vi "FGGA_Scroll_Pump_interface_server.vi"() -> ()   [LabVIEW 2014]
uses:
  <vilib>/NI/STM/TCP/TCP Write Options.ctl
  C:/Program Files (x86)/National Instruments/LabVIEW 2014/examples/Data Communication/Network Streams/Simple Network Streams/support/Network Stream Command.ctl
  <vilib>/Instr/_visa.llb/VISA Set IO Buffer Mask.ctl
  <vilib>/Platform/TimedLoop/XDataNode/timing_clust.ctl
  <vilib>/Platform/TimedLoop/XDataNode/nitl_modes.ctl
  <vilib>/Platform/TimedLoop/XDataNode/wakeup.ctl
  <vilib>/NI/STM/SubVIs/MetaDataElement.ctl
  <vilib>/NI/STM/TCP/Write Meta Data (TCP Ref).vi
  <vilib>/NI/STM/TCP/Get Connection Reference (TCP).vi
  <vilib>/Instr/_visa.llb/VISA Configure Serial Port (Instr).vi
  <vilib>/NI/STM/TCP/Write Meta Data (TCP Clst).vi
  <vilib>/NI/STM/TCP/Write Message (TCP).vi
  <vilib>/platform/TimedLoop/XDataNode/XDataNode.xnode
  <vilib>/Platform/TimedLoop/XDataNode/XDNodeRunTimeDep.lvlib
  <vilib>/NI/STM/NI STM.lvlib
panel:
  in  "options":T1={"ignore timeout error"=FALSE, "timeout ms (1000)"=1000}
  out "Standby Speed %\nDefault Set Value":u32=66 min=66 max=100
  out "error out 3":errorcluster
  out "Message Receive Array":string[](array[string])
  out "Scroll pump\nCommand":string[](array[string])
  out "Network Stream Error":errorcluster
  out "Standby Speed threshold":u32(slide) scale=66.0..100.0
  out "Normal Speed threshold":u32(slide) scale=50.0..100.0
  out "running?":bool
  out "Loop Count":i32
  in  "stop":bool
  out "Use Standby Speed":bool
  out "Serial / Pump Power cut error out":errorcluster
  in  "VISA resource name":refnum<visa-resource-name>="ASRL10::INSTR"
  out "Pump On/Off":bool
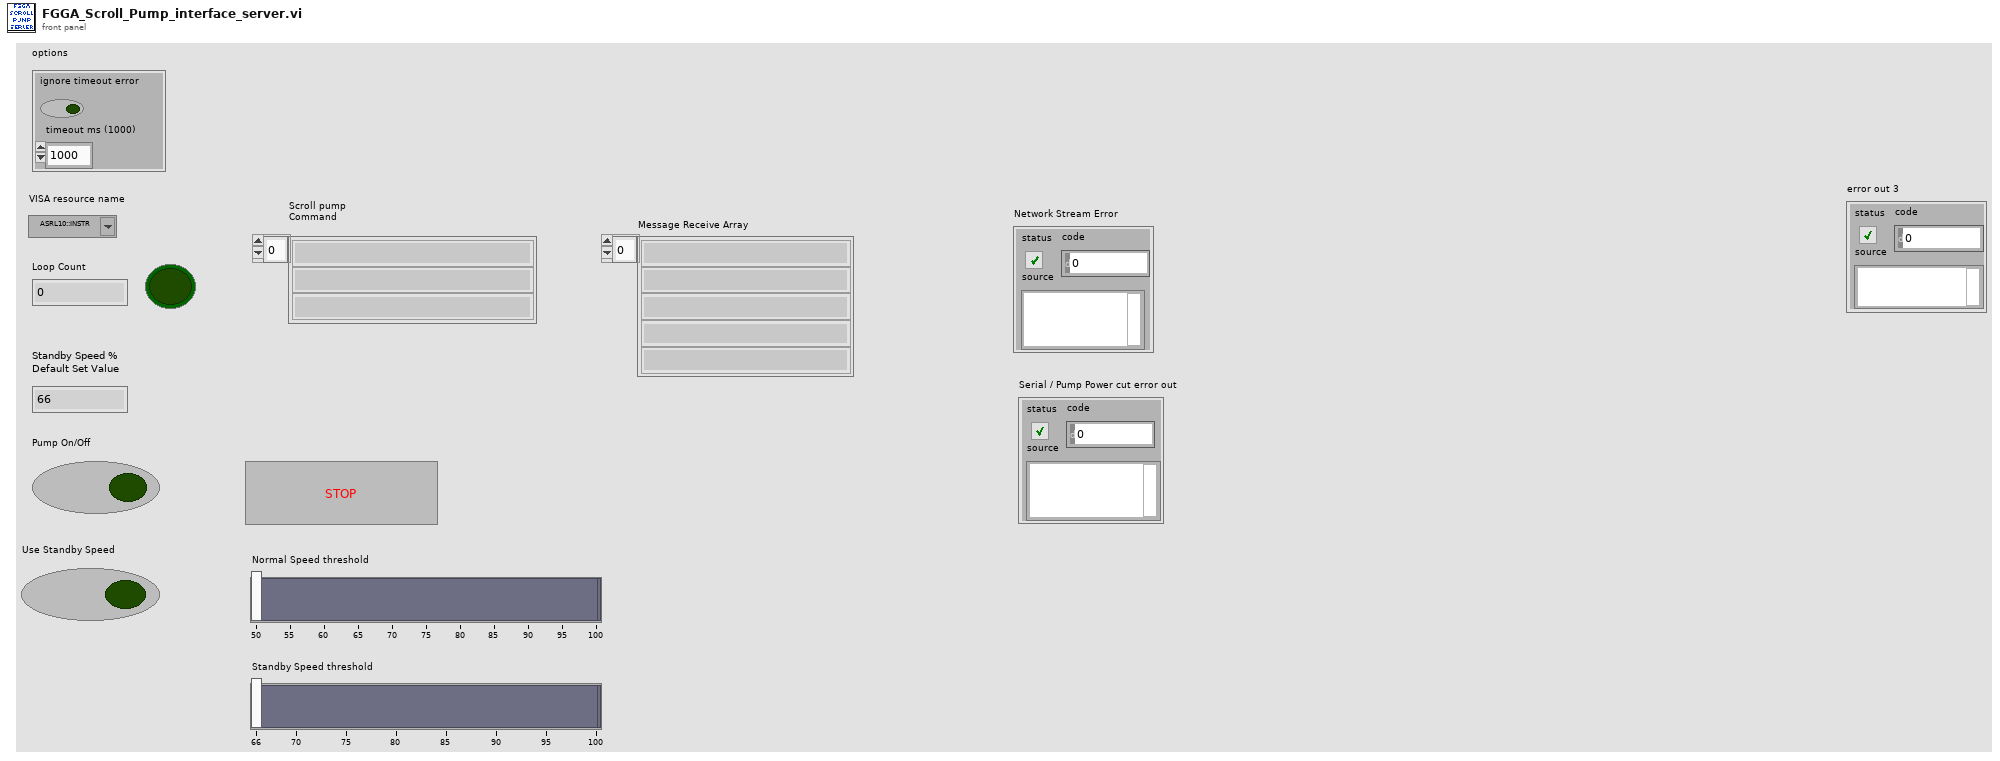
[diagram p1: front panel]
types:
  T1 = typedef "NI STM.lvlib/TCP Write Options.ctl" = cluster{"ignore timeout error":bool, "timeout ms (1000)":i32}
  T2 = typedef "XDNodeRunTimeDep.lvlib/timing_clust.ctl" = cluster{"Expected End [f-1]":u64, "Actual End [f-1]":u64, "Finished Late? [f-1]":bool, "Expected End [i-1]":u64, "Actual End [i-1]":u64, "Finished Late? [i-1]":bool, "Expected Start [i]":u64, "Actual Start [i]":u64, "Expected Start [f]":u64, "Actual Start [f]":u64, "Source Name":string, "Structure Name":string, "Period":i64, "Deadline":i64, "Offset":i64, "Start":i64, "Priority":i32, "Timeout":i32, "Mode":T3, "Wakeup Reason":T4, "Error":errorcluster, "Source Type":string, "Secondary Source Type":string, "Global End Time":u64, "Global Start Time":u64, "Frame Duration":u64, "Iteration Duration":u64, "Assigned CPU":i32, "I/O Scan Engine Mode":u32}
  T3 = typedef "XDNodeRunTimeDep.lvlib/nitl_modes.ctl" = enum32{"No Change", "Process missed periods, maintain original phase", "Discard missed periods, maintain original phase", "Process missed periods, ignore original phase", "Discard missed periods, ignore original phase"}
  T4 = typedef "XDNodeRunTimeDep.lvlib/wakeup.ctl" = enum32{"Normal", "Aborted", "Asynchronous wakeup", "Timing source error", "Timed loop error", "Timeout"}
  T5 = typedef "VISA Set IO Buffer Mask.ctl" = u16
  T6 = typedef "NI STM.lvlib/MetaDataElement.ctl" = string
  T7 = typedef "NI STM.lvlib/TCP Connection Info.ctl" = cluster{"connection ID":refnum<k5>, "meta data":T6[]}
  T8 = typedef "Network Stream Command.ctl" = cluster{"Message":string, "Message Data":variant}
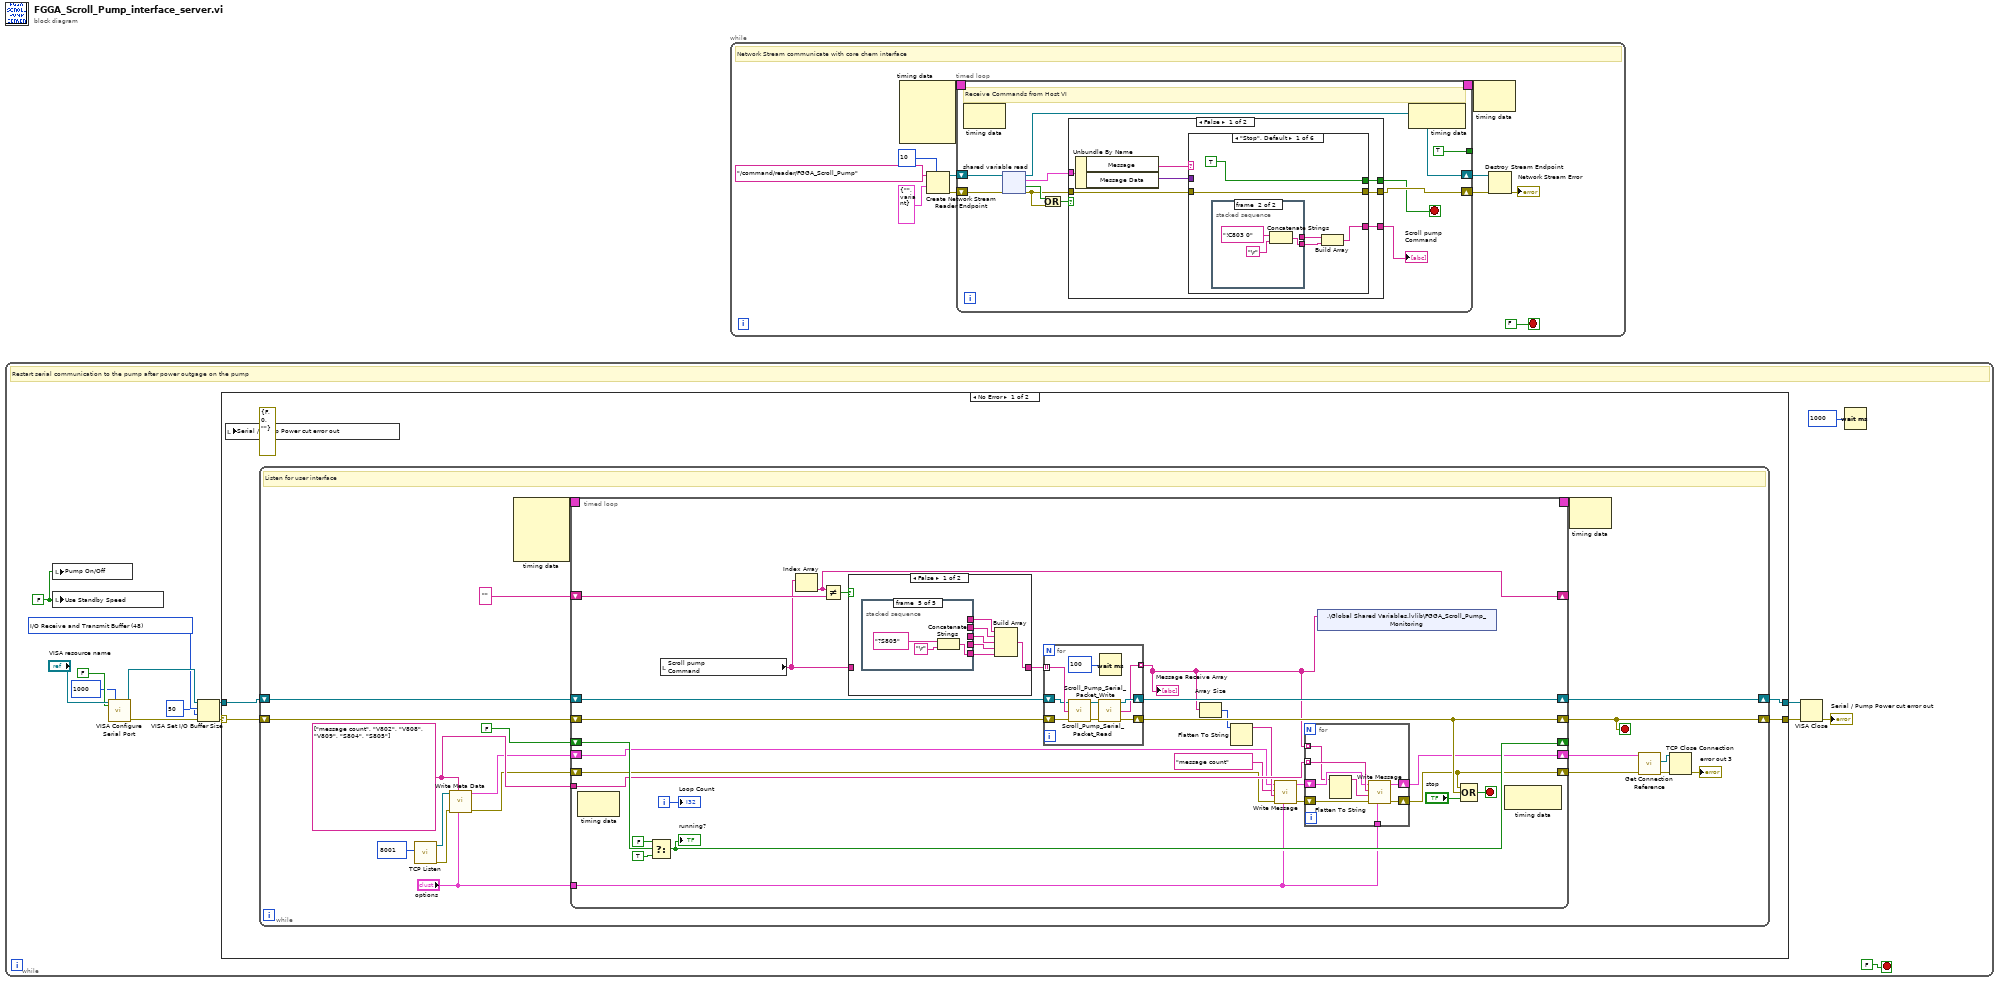
[diagram p0: block diagram]
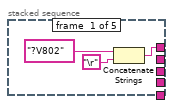
[diagram p2: hidden frame]
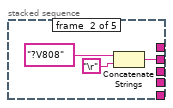
[diagram p3: hidden frame]
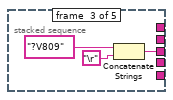
[diagram p4: hidden frame]
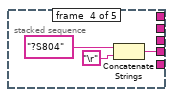
[diagram p5: hidden frame]
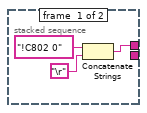
[diagram p8: hidden frame]
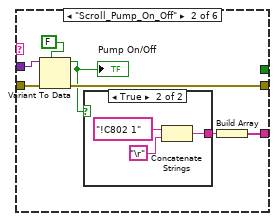
[diagram p9: hidden frame]
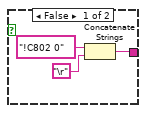
[diagram p10: hidden frame]
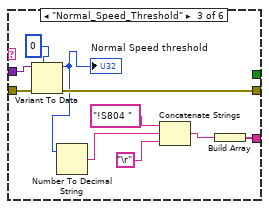
[diagram p11: hidden frame]
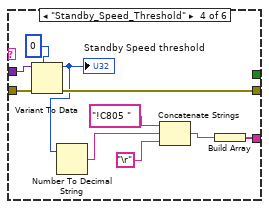
[diagram p12: hidden frame]
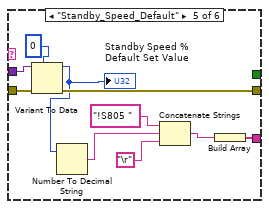
[diagram p13: hidden frame]
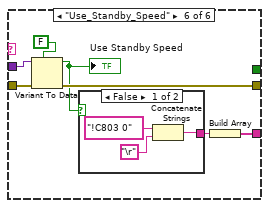
[diagram p14: hidden frame]
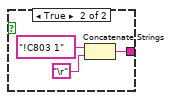
[diagram p15: hidden frame]
diagram:
  n1 = while {
    stop <- FALSE stop-if-true
    w2 = FALSE
    w11 = T5 48 items=["I/O Receive Buffer"=16, "I/O Transmit Buffer"=32, "I/O Receive and Transmit Buffer"=48] ("Mask")
    # "Restart serial communication to the pump after power outgage on the pump"
    n2 = local write "Pump On/Off"(w2) -> ()
    n3 = local write "Use Standby Speed"(w2) -> ()
    n4 = call-poly "VISA Configure Serial Port"("VISA resource name"="VISA resource name", "timeout (10sec)"=u32 1000, "Enable Termination\nChar (T)"=FALSE ("Enable Termination\nChar (T)")) -> ("VISA resource name out"=w12:refnum<visa-resource-name>, "error out"=w13:errorcluster)  [unwired: 11 in]
    n5 = VISA Set I/O Buffer Size(VISA resource name=w12, mask (16)=w11, size (4096)=u32 50, error in (no error)=w13) -> (VISA resource name out=w5:refnum<visa-resource-name>, error out=w4:errorcluster)
    n6 = case shown="No Error" w4 {
      selector: w4 -> [w20 w112]
      tunnel: w5 -> [w19 w113]
      tunnel: [w16 w113] -> w8
      tunnel: [w18 w112] -> w7
      frame No Error {
        n7 = local write "Serial / Pump Power cut error out"(errorcluster {"status"=FALSE, "code"=0, "source"=""} ("error out 2")) -> ()
        n8 = while {
          shift-right: [w22] -> w18
          shift-left: w20 -> [w37]
          shift-right: [w23] -> w16
          shift-left: w19 -> [w36]
          stop <- w22 stop-if-true
          w31 = T6[] ["message count", "V802", "V808", "V809", "S804", "S805"] ("meta data")
          # "Listen for user interface"
          n9 = call <vilib>:"TCP Listen.vi"("port"=u16 8001) -> ("error out"=w32:errorcluster, "connection ID"=w33:refnum<k5>)  [unwired: 6 in, 3 out]
          n10 = call-poly <vilib>:"Write Meta Data.vi"("options"="options", "meta data"=w31, "error in"=w32, "connection ID"=w33) -> ("error out"=w29:errorcluster, "connection info out"=w30:T7)  [unwired: 1 in, 5 out]
          n11 = node-c288() -> (w40:T2)  [unwired: 4 in]
          n12 = timed-loop {
            shift-right: [w64] -> _
            shift-left: FALSE -> [w67]
            shift-right: [w54] -> _
            shift-left: "" -> [w60]
            timing: w40 -> [_]
            timing-out: [_] -> w39
            tunnel: w31 -> [w53]
            shift-right: [w51] -> w23
            shift-left: w36 -> [w56]
            shift-right: [w62] -> w22
            shift-left: w37 -> [w55]
            shift-right: [w52] -> w25
            shift-left: w30 -> [w47]
            shift-right: [w50] -> w24
            shift-left: w29 -> [w48]
            tunnel: "options" -> [w41]
            i -> [w68]
            stop <- w61 stop-if-true
            n13 = node-c288() -> ()  [unwired: 1 in, 1 out]
            n14 = Select(t=FALSE, s=w67, f=TRUE) -> (s? t:f=w64:bool)
            "running?" <- w64
            n15 = local read "Scroll pump\nCommand"() -> (w58:string[])
            n16 = Index Array(array=w58) -> (element=w54:string)  [unwired: 1 in]
            n17 = Not Equal?(x=w54, y=w60) -> (x != y?=w59:bool)
            n18 = case shown="False" w59 {
              tunnel: [w81 w100] -> w57
              tunnel: w58 -> [_ w100]
              frame False {
                n19 = stacked-sequence {
                  tunnel: [w85 _ _ _ _] -> w82
                  tunnel: [_ w88 _ _ _] -> w83
                  tunnel: [_ _ w91 _ _] -> w84
                  tunnel: [_ _ _ w94 _] -> w80
                  tunnel: [_ _ _ _ w97] -> w79
                  frame #0 {
                    n20 = Concatenate Strings("?V802" ("string"), "\r") -> (w85:string)
                  }
                  frame #1 {
                    n21 = Concatenate Strings("?V808" ("string"), "\r") -> (w88:string)
                  }
                  frame #2 {
                    n22 = Concatenate Strings("?V809" ("string"), "\r") -> (w91:string)
                  }
                  frame #3 {
                    n23 = Concatenate Strings("?S804" ("string"), "\r") -> (w94:string)
                  }
                  frame #4 {
                    n24 = Concatenate Strings("?S805" ("string"), "\r") -> (w97:string)
                  }
                }
                n25 = Build Array(w82, w83, w84, w80, w79) -> (w81:string[])
              }
              frame True {
              }
            }
            n26 = for {
              tunnel: [w107] -> w42 mode=indexing
              tunnel: w57 -> [w106] mode=indexing
              shift-right: [w109] -> w51
              shift-left: w56 -> [w105]
              shift-right: [w108] -> w62
              shift-left: w55 -> [w104]
              n27 = call "Scroll_Pump_Serial_Packet_Write.vi"("VISA resource name In"=w105, "Data in"=w106, "error in (no error)"=w104) -> ("VISA resource name Out"=w103:refnum<visa-resource-name>, "error out"=w102:errorcluster)  [unwired: 11 in]
              n28 = call "Scroll_Pump_Serial_Packet_Read.vi"("VISA resource In"=w103, "error in"=w102) -> ("VISA resource Out"=w109:refnum<visa-resource-name>, "Data Out"=w107:string, "error out"=w108:errorcluster)  [unwired: 11 in]
              n29 = Wait (ms)(milliseconds to wait=u32 100) -> ()  [unwired: 1 out]
            }
            "Message Receive Array" <- w42
            n30 = Array Size(array=w42) -> (size(s)=w44:i32)
            n31 = Flatten To String(anything=w44) -> (data string=w49:string)  [unwired: 1 in, 4 out]
            n32 = call-poly <vilib>:"Write Message.vi"("options"=w41, "error in"=w48, "data"=w49, "name"="message count", "connection info in"=w47) -> ("error out"=w45:errorcluster, "connection info out"=w46:T7)  [unwired: 5 out]
            n33 = for {
              tunnel: w42 -> [w71] mode=indexing
              tunnel: w53 -> [w76] mode=indexing
              shift-right: [w72] -> w52
              shift-left: w46 -> [w75]
              shift-right: [w73] -> w50
              shift-left: w45 -> [w74]
              tunnel: w41 -> [w69]
              n34 = Flatten To String(anything=w71) -> (data string=w70:string)  [unwired: 1 in, 4 out]
              n35 = call-poly <vilib>:"Write Message.vi"("options"=w69, "error in"=w74, "data"=w70, "name"=w76, "connection info in"=w75) -> ("error out"=w73:errorcluster, "connection info out"=w72:T7)  [unwired: 5 out]
            }
            n36 = shared-variable ".\\Global Shared Variables.lvlib\\FGGA_Scroll_Pump_Monitoring"(w42) -> ()  [unwired: 1 in, 1 out]
            n37 = Compound Arithmetic op=OR(w50, w62, "stop") -> (w61:bool)
            n38 = node-c288() -> ()  [unwired: 1 in, 1 out]
            "Loop Count" <- w68
          }
          n39 = node-c288(w39) -> ()  [unwired: 1 out]
          n40 = call-poly <vilib>:"Get Connection Reference.vi"("error in"=w24, "connection info in"=w25) -> ("error out"=w28:errorcluster, "connection ID out"=w27:refnum<k5>)  [unwired: 8 out]
          n41 = TCP Close Connection(connection ID=w27, error in (no error)=w28) -> (error out=→"error out 3":errorcluster)  [unwired: 2 out]
        }
      }
      frame Error {
      }
    }
    n42 = VISA Close(VISA resource name=w8, error in (no error)=w7) -> (error out=→"Serial / Pump Power cut error out":errorcluster)
    n43 = Wait (ms)(milliseconds to wait=u32 1000) -> ()  [unwired: 1 out]
  }
  n44 = while {
    stop <- FALSE stop-if-true
    # "Network Stream communicate with core chem interface"
    n45 = node-c288() -> (w115:T2)  [unwired: 4 in]
    n46 = Create Network Stream Reader Endpoint(7:10 ("reader buffer size"), 9:T8 {"Message"="", "Message Data"=variant} ("Message Cluster"), 11:"/command/reader/FGGA_Scroll_Pump" ("reader url")) -> (0:w120:errorcluster, 3:w121:refnum<k21>)  [unwired: 4 in]
    n47 = timed-loop "Host->Target Command Reader" {
      shift-right: [w126] -> w118
      shift-left: w120 -> [w135]
      shift-right: [w133] -> w117
      shift-left: w121 -> [w134]
      tunnel: [TRUE] -> _
      timing: w115 -> [_]
      timing-out: [_] -> w114
      stop <- w125 stop-if-true
      # "Receive Commands from Host VI"
      n48 = node-c288() -> ()  [unwired: 1 in, 1 out]
      n49 = shared-variable-read(w134, w135) -> (w133:refnum<k21>, w129:errorcluster, w131:bool, w132:T8)  [unwired: 1 in]
      n50 = Or(x=w131, y=w129) -> (x .or. y?=w130:bool)
      n51 = case shown="False" w130 {
        selector: w130 -> [_ w212]
        tunnel: w129 -> [w144 w213]
        tunnel: [w143 w213] -> w126
        tunnel: w132 -> [w141 _]
        tunnel: [w142 w212] -> w125
        tunnel: [w138 _] -> w127
        frame False {
          n52 = Unbundle By Name(w141) -> ("Message"=w140:string, "Message Data"=w139:variant)
          n53 = case shown="\"Stop\", Default" w140 {
            tunnel: w144 -> [w149 w162 w178 w188 w198 w205]
            tunnel: [w149 w161 w177 w187 w197 w204] -> w143
            tunnel: w139 -> [_ w160 w176 w186 w196 w203]
            tunnel: [TRUE _ _ _ _ _] -> w142
            tunnel: [w145 w156 w170 w180 w190 w199] -> w138
            frame "Stop", Default {
              n54 = stacked-sequence {
                tunnel: [w150 _] -> w147
                tunnel: [_ w153] -> w146
                frame #0 {
                  n55 = Concatenate Strings("!C802 0" ("string"), "\r") -> (w150:string)
                }
                frame #1 {
                  n56 = Concatenate Strings("!C803 0" ("string"), "\r") -> (w153:string)
                }
              }
              n57 = Build Array(w147, w146) -> (w145:string[])
            }
            frame "Scroll_Pump_On_Off" {
              n58 = Variant To Data(error in=w162, type=FALSE, Variant=w160) -> (data=w158:bool, error out=w161:errorcluster)
              "Pump On/Off" <- w158
              n59 = case shown="True" w158 {
                tunnel: [w163 w166] -> w157
                frame False {
                  n60 = Concatenate Strings("!C802 0" ("string"), "\r") -> (w163:string)
                }
                frame True {
                  n61 = Concatenate Strings("!C802 1" ("string"), "\r") -> (w166:string)
                }
              }
              n62 = Build Array(w157) -> (w156:string[])
            }
            frame "Normal_Speed_Threshold" {
              n63 = Variant To Data(error in=w178, type=u32 0, Variant=w176) -> (data=w169:u32, error out=w177:errorcluster)
              "Normal Speed threshold" <- w169
              n64 = Number To Decimal String(number=w169) -> (decimal integer string=w172:string)  [unwired: 1 in]
              n65 = Concatenate Strings("!S804 " ("string"), w172, "\r") -> (w171:string)
              n66 = Build Array(w171) -> (w170:string[])
            }
            frame "Standby_Speed_Threshold" {
              n67 = Variant To Data(error in=w188, type=u32 0, Variant=w186) -> (data=w179:u32, error out=w187:errorcluster)
              "Standby Speed threshold" <- w179
              n68 = Number To Decimal String(number=w179) -> (decimal integer string=w182:string)  [unwired: 1 in]
              n69 = Concatenate Strings("!C805 " ("string"), w182, "\r") -> (w181:string)
              n70 = Build Array(w181) -> (w180:string[])
            }
            frame "Standby_Speed_Default" {
              n71 = Variant To Data(error in=w198, type=u32 0, Variant=w196) -> (data=w189:u32, error out=w197:errorcluster)
              "Standby Speed %\nDefault Set Value" <- w189
              n72 = Number To Decimal String(number=w189) -> (decimal integer string=w192:string)  [unwired: 1 in]
              n73 = Concatenate Strings("!S805 " ("string"), w192, "\r") -> (w191:string)
              n74 = Build Array(w191) -> (w190:string[])
            }
            frame "Use_Standby_Speed" {
              n75 = Variant To Data(error in=w205, type=FALSE, Variant=w203) -> (data=w201:bool, error out=w204:errorcluster)
              "Use Standby Speed" <- w201
              n76 = case shown="False" w201 {
                tunnel: [w206 w209] -> w200
                frame False {
                  n77 = Concatenate Strings("!C803 0" ("string"), "\r") -> (w206:string)
                }
                frame True {
                  n78 = Concatenate Strings("!C803 1" ("string"), "\r") -> (w209:string)
                }
              }
              n79 = Build Array(w200) -> (w199:string[])
            }
          }
        }
        frame True {
        }
      }
      "Scroll pump\nCommand" <- w127
      n80 = node-c288() -> ()  [unwired: 1 in, 1 out]
    }
    n81 = node-c288(w114) -> ()  [unwired: 1 out]
    n82 = Destroy Stream Endpoint(8:w118, 11:w117) -> (0:→"Network Stream Error":errorcluster)
  }
